vi "ConfigureAdaptorr05.vi"() -> ()   [LabVIEW 2011]
panel:
  in  "Trip Point 1(Torr)":dbl=700.0
  in  "Set Point D (Torr)":dbl=40.0
  in  "Set Point C (Torr)":dbl=20.0
  in  "Set Point B (Torr)":dbl=76.0
  in  "Set Point A (Torr)":dbl=10.0
  in  "Trip Point 2 (Torr)":dbl=200.0
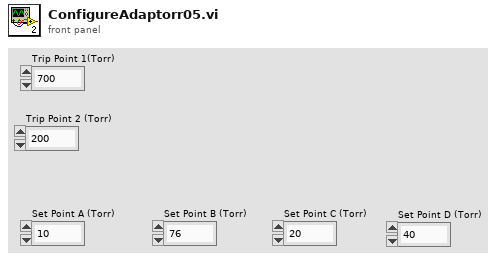
[diagram p1: front panel]
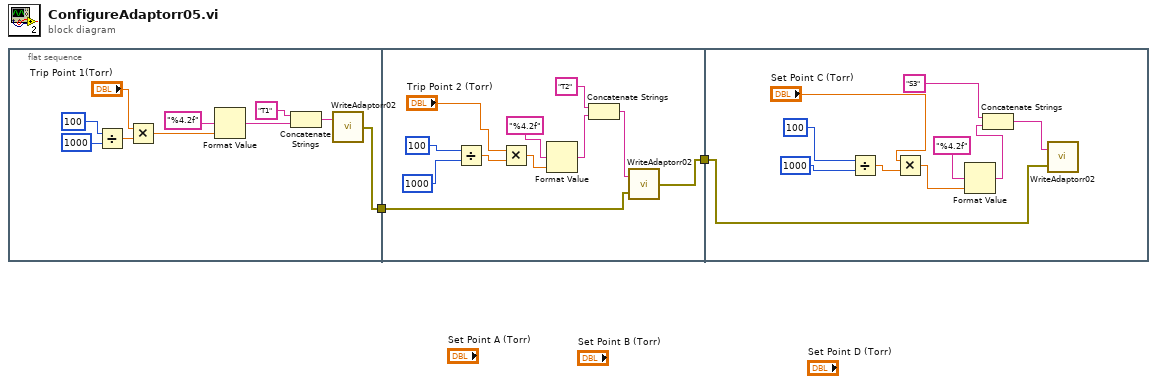
[diagram p0: block diagram]
diagram:
  n1 = flat-sequence {
    tunnel: [w5] -> w1
    tunnel: [w16] -> w2
    tunnel: w1 -> [w18]
    tunnel: w2 -> [w27]
    frame #0 {
      n2 = Divide(x=100, y=1000) -> (x/y=w10:dbl)
      n3 = Multiply(x="Trip Point 1(Torr)", y=w10) -> (x*y=w4:dbl)
      n4 = Format Value(format string="%4.2f", value (0)=w4) -> (output string=w7:string)  [unwired: 1 in]
      n5 = Concatenate Strings("T1", w7) -> (w6:string)
      n6 = call "WriteAdaptorr02.vi"("string to write"=w6) -> ("error out"=w5:errorcluster)  [unwired: 1 in]
    }
    frame #1 {
      n7 = Divide(x=100, y=1000) -> (x/y=w21:dbl)
      n8 = Multiply(x="Trip Point 2 (Torr)", y=w21) -> (x*y=w15:dbl)
      n9 = Format Value(format string="%4.2f", value (0)=w15) -> (output string=w13:string)  [unwired: 1 in]
      n10 = Concatenate Strings("T2", w13) -> (w17:string)
      n11 = call "WriteAdaptorr02.vi"("error in (no error)"=w18, "string to write"=w17) -> ("error out"=w16:errorcluster)
    }
    frame #2 {
      n12 = Divide(x=100, y=1000) -> (x/y=w31:dbl)
      n13 = Multiply(x="Set Point C (Torr)", y=w31) -> (x*y=w25:dbl)
      n14 = Format Value(format string="%4.2f", value (0)=w25) -> (output string=w24:string)  [unwired: 1 in]
      n15 = Concatenate Strings("S3", w24) -> (w28:string)
      n16 = call "WriteAdaptorr02.vi"("error in (no error)"=w27, "string to write"=w28) -> ()  [unwired: 1 out]
    }
  }
